vi "datahandle.vi"(8 "error in (no error)":errorcluster caption="错误输入（无错误）", 10 "data":string[][](array[string]), 11 "HJ212 输入":refnum<class "HJ212.lvclass">) -> (0 "error out":errorcluster caption="错误输出", 2 "message":string, 3 "HJ212 输出":refnum<class "HJ212.lvclass">)   [LabVIEW 2016, in "潮位站数据传输.lvlib" / "HJ212.lvclass"]
uses:
  HJ212.lvclass
  data_combination/data_combination.lvclass/data_combination.ctl
  data_combination/data_combination.lvclass
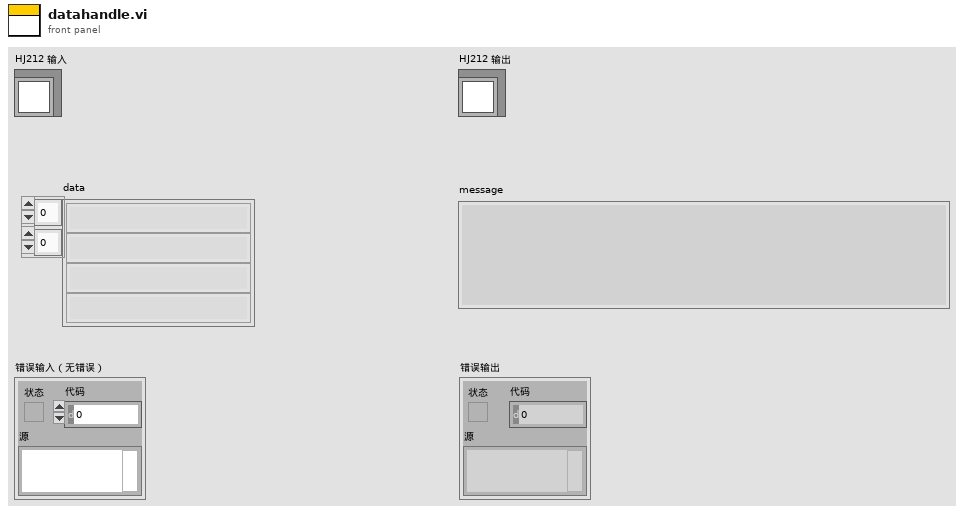
[diagram p1: front panel]
types:
  T1 = cluster{"请求编码QN(20)":string, "系统编码ST(5)":string, "命令编码CN(7)":string, "访问密码PW(9)":string, "设备唯一标识MN(27)":string, "拆分包及应答标志FLAG(8)":string, "总包数PNUM(9)":string, "包号PNO(8)":string, "指令参数CP(0-950)":string}
  T2 = typedef "潮位站数据传输.lvlib/table.ctl" = string
  T3 = typedef "潮位站数据传输.lvlib/Type.ctl" = string
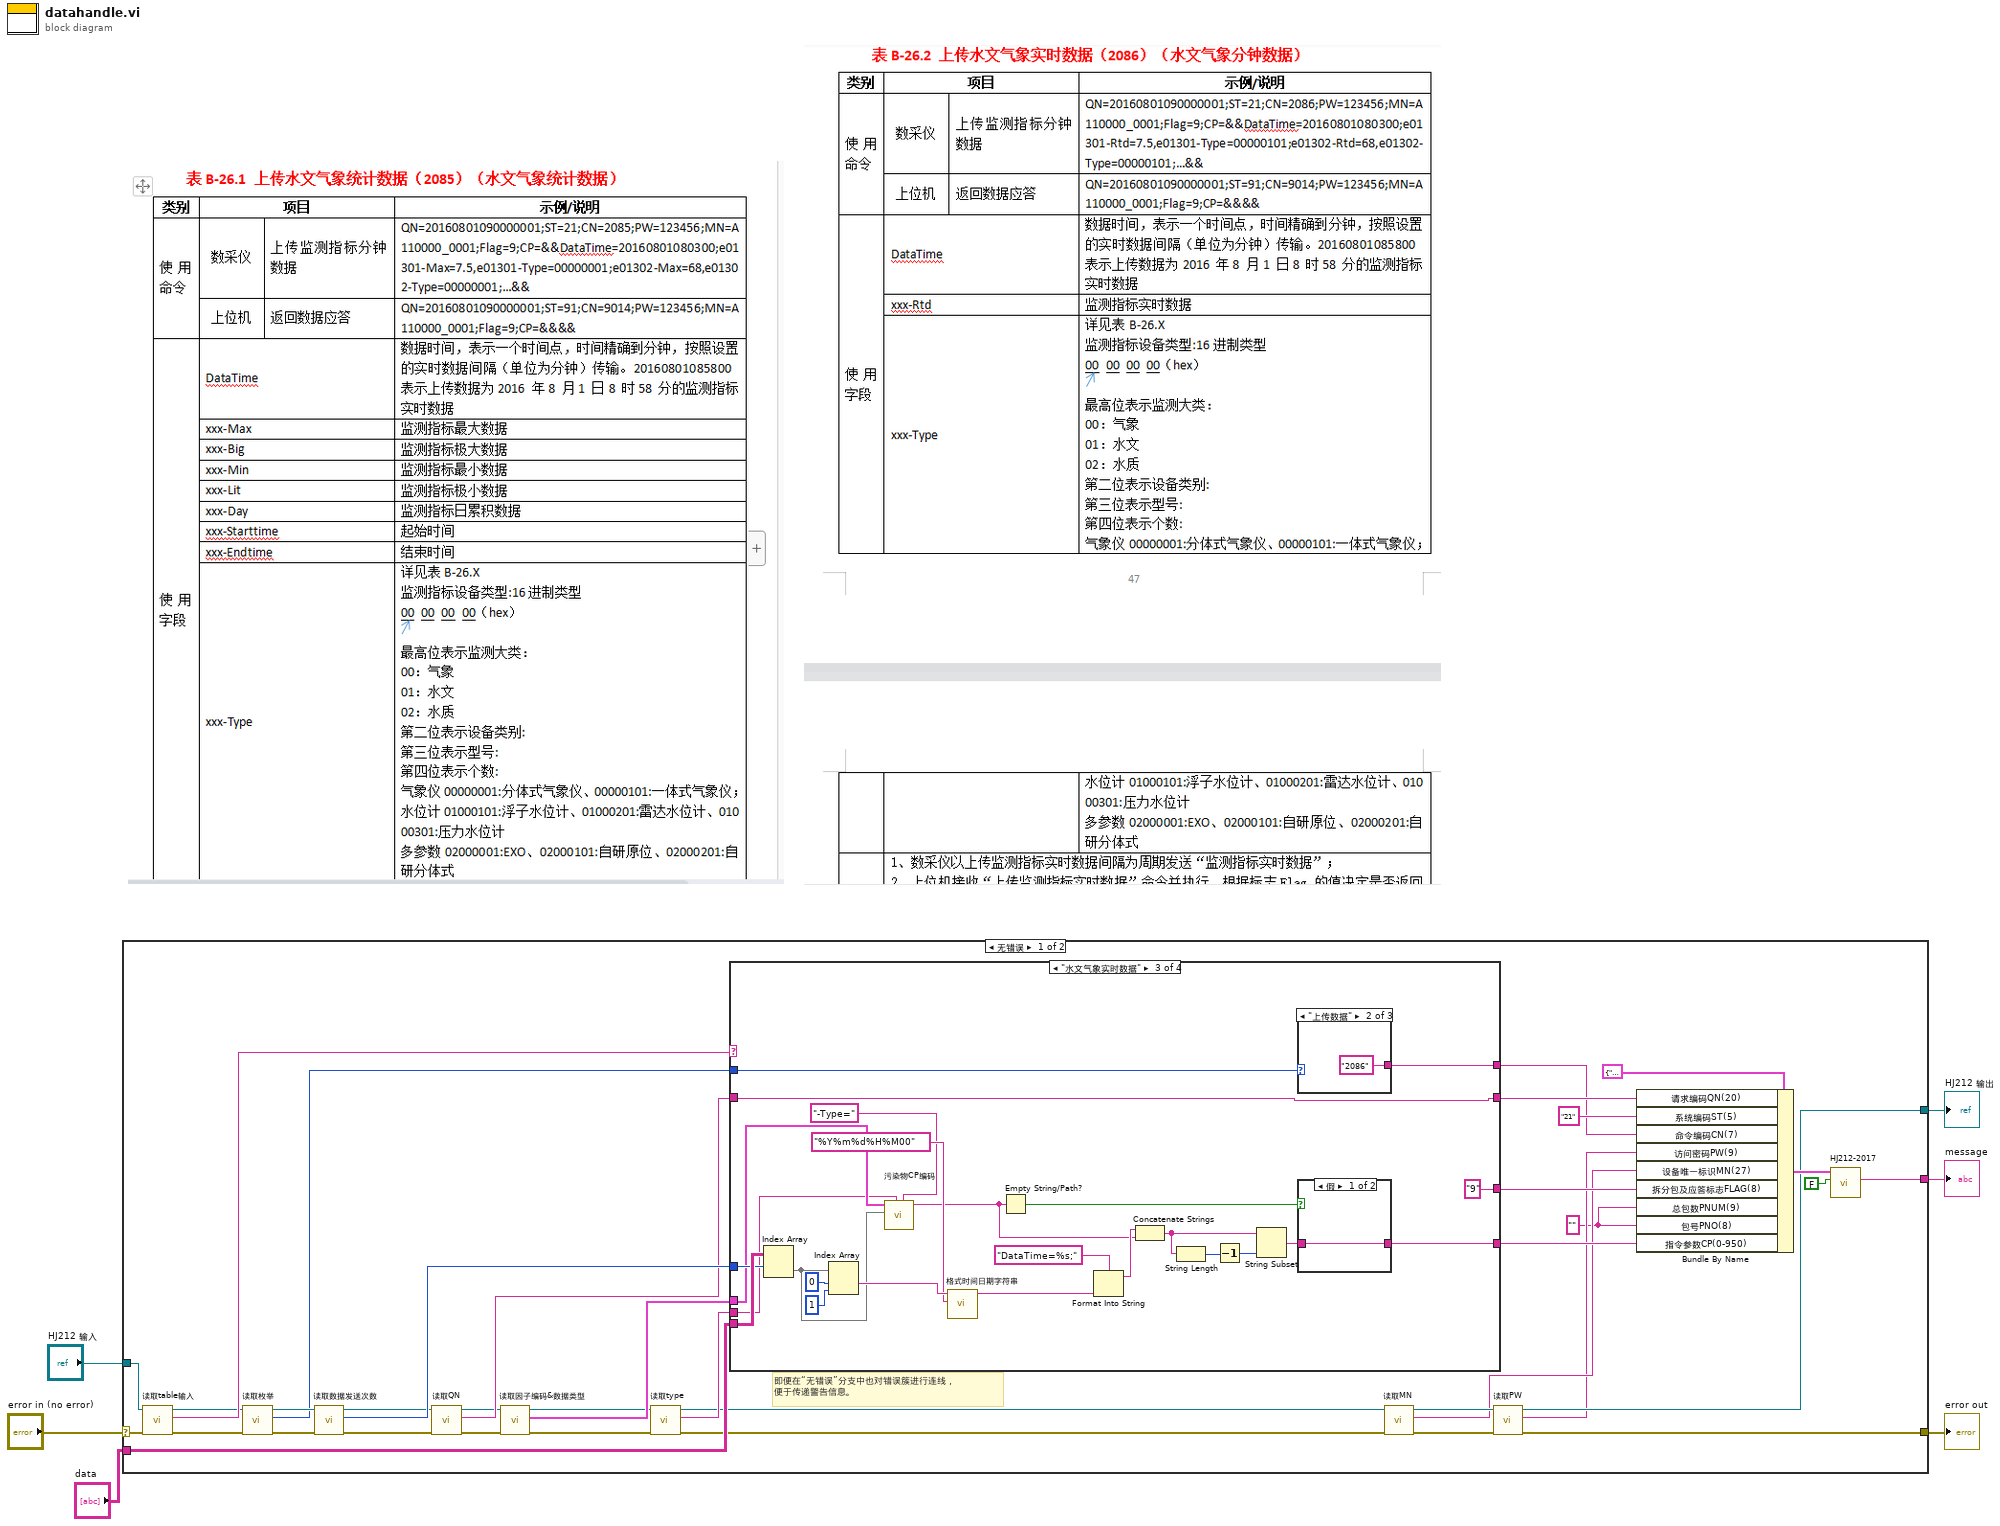
[diagram p0: block diagram]
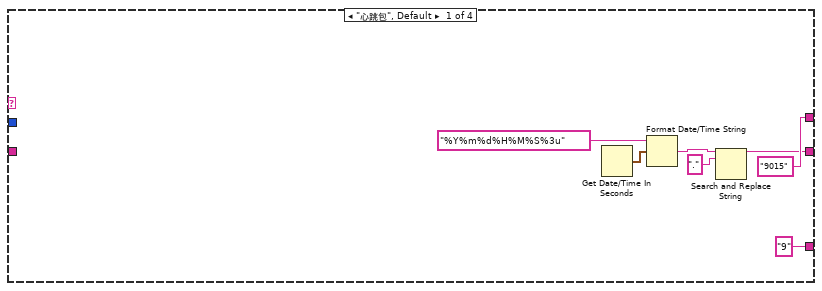
[diagram p2: hidden frame]
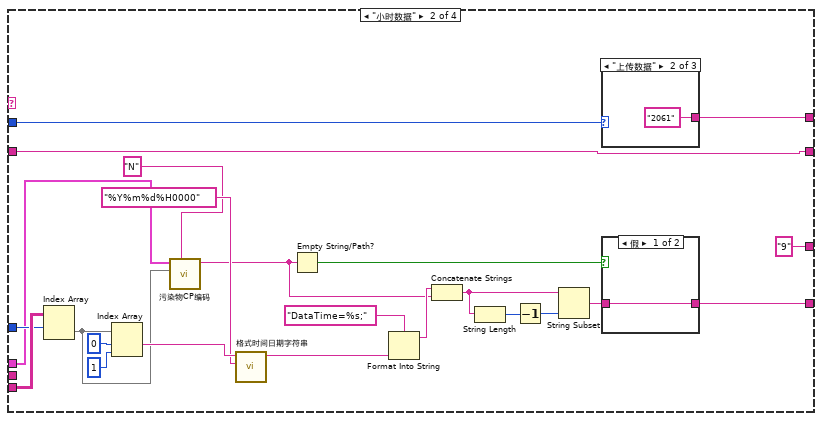
[diagram p3: hidden frame]
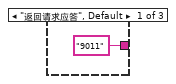
[diagram p4: hidden frame]
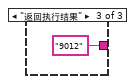
[diagram p5: hidden frame]
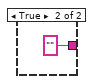
[diagram p6: hidden frame]
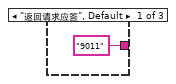
[diagram p7: hidden frame]
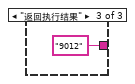
[diagram p8: hidden frame]
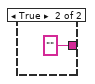
[diagram p9: hidden frame]
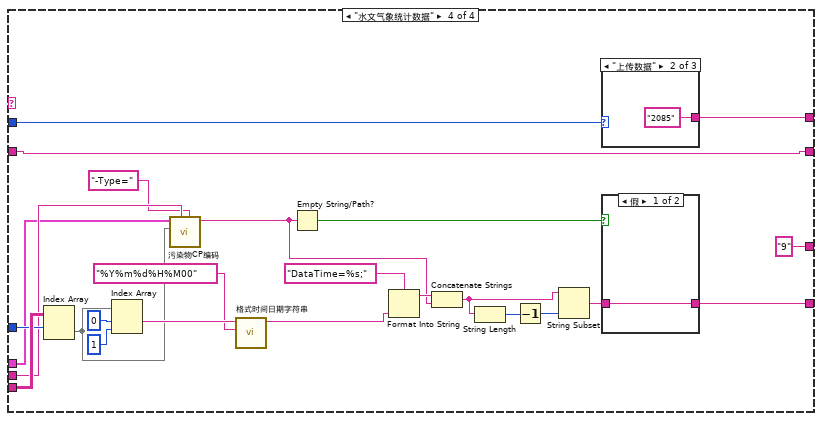
[diagram p10: hidden frame]
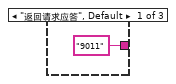
[diagram p11: hidden frame]
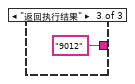
[diagram p12: hidden frame]
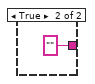
[diagram p13: hidden frame]
diagram:
  n1 = case shown="无错误" "error in (no error)" {
    selector: "error in (no error)" -> [w17 w138]
    tunnel: [w16 w138] -> w5
    tunnel: [w24 w137] -> w3
    tunnel: "HJ212 输入" -> [w26 w137]
    tunnel: [w43 _] -> w2
    tunnel: "data" -> [w36 _]
    frame No Error {
      w15 = "" ("总包数PNUM(9)")
      # "即便在“无错误”分支中也对错误簇进行连线，\n便于传递警告信息。"
      n2 = call "读取table输入.vi"("error in (no error)"=w17, "data_combination输入"=w26) -> ("error out"=w21:errorcluster, "table输入"=w39:T2, "data_combination输出"=w38:refnum<class "HJ212.lvclass">)  [unwired: 7 in]
      n3 = call "读取枚举.vi"("error in (no error)"=w21, "data_combination输入"=w38) -> ("error out"=w20:errorcluster, "枚举"=w28:enum16{"返回请求应答", "上传数据", "返回执行结果"}, "data_combination输出"=w37:refnum<class "HJ212.lvclass">)  [unwired: 7 in]
      n4 = call "读取数据发送次数.vi"("error in (no error)"=w20, "data_combination输入"=w37) -> ("error out"=w19:errorcluster, "数据发送次数"=w35:i32, "data_combination输出"=w31:refnum<class "HJ212.lvclass">)  [unwired: 7 in]
      n5 = call "读取QN.vi"("error in (no error)"=w19, "data_combination输入"=w31) -> ("error out"=w13:errorcluster, "QN"=w30:string, "data_combination输出"=w14:refnum<class "HJ212.lvclass">)  [unwired: 7 in]
      n6 = call "读取因子编码&数据类型.vi"("error in (no error)"=w13, "data_combination输入"=w14) -> ("error out"=w7:errorcluster, "因子编码&数据类型"=w12:cluster{"因子编码":string, "数据类型":string}[], "data_combination输出"=w8:refnum<class "HJ212.lvclass">)  [unwired: 7 in]
      n7 = call "读取type.vi"("error in (no error)"=w7, "data_combination输入"=w8) -> ("error out"=w9:errorcluster, "type"=w11:T3, "data_combination输出"=w10:refnum<class "HJ212.lvclass">)  [unwired: 7 in]
      n8 = case shown="\"水文气象实时数据\"" w39 {
        tunnel: w36 -> [_ w72 w101 w115]
        tunnel: w35 -> [_ w71 w100 w112]
        tunnel: [_ w61 w90 w114] -> w34
        tunnel: ["9" ("ST") "9" ("ST") "9" ("ST") "9" ("ST")] -> w33
        tunnel: [w46 w59 w88 w116] -> w29
        tunnel: w30 -> [_ w59 w88 w116]
        tunnel: w28 -> [_ w58 w87 w118]
        tunnel: ["9015" ("ST") w57 w86 w117] -> w27
        tunnel: w12 -> [_ w54 w84 w109]
        tunnel: w11 -> [_ _ w79 w111]
        frame "心跳包", Default {
          n9 = Get Date/Time In Seconds() -> (seconds since 1Jan1904=w49:timestamp)
          n10 = Format Date/Time String(time format string (%c)="%Y%m%d%H%M%S%3u" ("时间格式字符串(%c)"), seconds (now)=w49) -> (date/time string=w48:string)  [unwired: 1 in]
          n11 = Search and Replace String(input string=w48, search string="." ("搜索字符串")) -> (result string=w46:string)  [unwired: 6 in, 3 out]
        }
        frame "小时数据" {
          n12 = Index Array(array=w72, index (row)=w71) -> (element=w51:string[])  [unwired: 1 in]
          n13 = Index Array(array=w51, index #1=0 ("索引"), index #2=1 ("索引")) -> (element #1=w70:string)  [unwired: 1 out]
          n14 = call "污染物CP编码.vi"("Type/标识"="N" ("字符串"), "污染物浓度"=w51, "因子编码&数据类型"=w54) -> ("编码输出"=w52:string)  [unwired: 8 in]
          n15 = call "格式时间日期字符串.vi"("时间格式字符串(%c)"="%Y%m%d%H0000", "字符串"=w70) -> ("result string"=w67:string)  [unwired: 9 in]
          n16 = Empty String/Path?(string/path=w52) -> (empty?=w53:bool)
          n17 = Format Into String(format string="DataTime=%s;", w67) -> (resulting string=w62:string)  [unwired: 2 in, 1 out]
          n18 = Concatenate Strings(w62, w52) -> (w64:string)
          n19 = String Length(string=w64) -> (length=w66:i32)
          n20 = Decrement(x=w66) -> (x-1=w65:i32)
          n21 = String Subset(string=w64, length (rest)=w65) -> (substring=w63:string)  [unwired: 1 in]
          n22 = case shown="\"上传数据\"" w58 {
            tunnel: ["9011" ("CN") "2061" ("CN") "9012" ("CN")] -> w57
            frame "返回请求应答", Default {
            }
            frame "上传数据" {
            }
            frame "返回执行结果" {
            }
          }
          n23 = case shown="假" w53 {
            tunnel: [w77 ""] -> w61
            tunnel: w63 -> [w77 _]
            frame False {
            }
            frame True {
            }
          }
        }
        frame "水文气象实时数据" {
          n24 = Index Array(array=w101, index (row)=w100) -> (element=w81:string[])  [unwired: 1 in]
          n25 = Index Array(array=w81, index #1=0 ("索引"), index #2=1 ("索引")) -> (element #1=w99:string)  [unwired: 1 out]
          n26 = call "污染物CP编码.vi"("-flag="="-Type=" ("-fag="), "Type/标识"=w79, "污染物浓度"=w81, "因子编码&数据类型"=w84) -> ("编码输出"=w82:string)  [unwired: 7 in]
          n27 = call "格式时间日期字符串.vi"("时间格式字符串(%c)"="%Y%m%d%H%M00", "字符串"=w99) -> ("result string"=w96:string)  [unwired: 9 in]
          n28 = Empty String/Path?(string/path=w82) -> (empty?=w83:bool)
          n29 = Format Into String(format string="DataTime=%s;", w96) -> (resulting string=w91:string)  [unwired: 2 in, 1 out]
          n30 = Concatenate Strings(w91, w82) -> (w93:string)
          n31 = String Length(string=w93) -> (length=w95:i32)
          n32 = Decrement(x=w95) -> (x-1=w94:i32)
          n33 = String Subset(string=w93, length (rest)=w94) -> (substring=w92:string)  [unwired: 1 in]
          n34 = case shown="\"上传数据\"" w87 {
            tunnel: ["9011" ("CN") "2086" ("CN") "9012" ("CN")] -> w86
            frame "返回请求应答", Default {
            }
            frame "上传数据" {
            }
            frame "返回执行结果" {
            }
          }
          n35 = case shown="假" w83 {
            tunnel: [w106 ""] -> w90
            tunnel: w92 -> [w106 _]
            frame False {
            }
            frame True {
            }
          }
        }
        frame "水文气象统计数据" {
          n36 = Index Array(array=w115, index (row)=w112) -> (element=w108:string[])  [unwired: 1 in]
          n37 = Index Array(array=w108, index #1=0 ("索引"), index #2=1 ("索引")) -> (element #1=w130:string)  [unwired: 1 out]
          n38 = call "污染物CP编码.vi"("-flag="="-Type=" ("-fag="), "Type/标识"=w111, "污染物浓度"=w108, "因子编码&数据类型"=w109) -> ("编码输出"=w119:string)  [unwired: 7 in]
          n39 = call "格式时间日期字符串.vi"("时间格式字符串(%c)"="%Y%m%d%H%M00", "字符串"=w130) -> ("result string"=w127:string)  [unwired: 9 in]
          n40 = Empty String/Path?(string/path=w119) -> (empty?=w120:bool)
          n41 = Format Into String(format string="DataTime=%s;", w127) -> (resulting string=w122:string)  [unwired: 2 in, 1 out]
          n42 = Concatenate Strings(w122, w119) -> (w124:string)
          n43 = String Length(string=w124) -> (length=w126:i32)
          n44 = Decrement(x=w126) -> (x-1=w125:i32)
          n45 = String Subset(string=w124, length (rest)=w125) -> (substring=w123:string)  [unwired: 1 in]
          n46 = case shown="\"上传数据\"" w118 {
            tunnel: ["9011" ("CN") "2085" ("CN") "9012" ("CN")] -> w117
            frame "返回请求应答", Default {
            }
            frame "上传数据" {
            }
            frame "返回执行结果" {
            }
          }
          n47 = case shown="假" w120 {
            tunnel: [w135 ""] -> w114
            tunnel: w123 -> [w135 _]
            frame False {
            }
            frame True {
            }
          }
        }
      }
      n48 = call "读取MN.vi"("error in (no error)"=w9, "data_combination输入"=w10) -> ("error out"=w18:errorcluster, "MN"=w23:string, "data_combination输出"=w25:refnum<class "HJ212.lvclass">)  [unwired: 7 in]
      n49 = call "读取PW.vi"("error in (no error)"=w18, "data_combination输入"=w25) -> ("error out"=w16:errorcluster, "PW"=w22:string, "data_combination输出"=w24:refnum<class "HJ212.lvclass">)  [unwired: 7 in]
      n50 = Bundle By Name(cluster=T1 {"请求编码QN(20)"="", "系统编码ST(5)"="", "命令编码CN(7)"="", "访问密码PW(9)"="", "设备唯一标识MN(27)"="", "拆分包及应答标志FLAG(8)"="", "总包数PNUM(9)"="", "包号PNO(8)"="", "指令参数CP(0-950)"=""} ("数据段"), "请求编码QN(20)"=w29, "系统编码ST(5)"="21", "命令编码CN(7)"=w27, "访问密码PW(9)"=w22, "设备唯一标识MN(27)"=w23, "拆分包及应答标志FLAG(8)"=w33, "总包数PNUM(9)"=w15, "包号PNO(8)"=w15, "指令参数CP(0-950)"=w34) -> (w40:T1)
      n51 = call "HJ212-2017.vi"("PWD？"=FALSE, "数据段"=w40) -> ("通讯包字符串"=w43:string)  [unwired: 7 in, 2 out]
    }
    frame Error {
    }
  }
  "error out" <- w5
  "HJ212 输出" <- w3
  "message" <- w2
